vi "面积.vi"(8 "error in (no error)":errorcluster caption="错误输入（无错误）", 11 "矩形类 输入":refnum<class "矩形.lvclass"> caption="DNL_LabVIEW Object in") -> (0 "error out":errorcluster caption="错误输出", 2 "面积":dbl, 3 "矩形类 输出":refnum<class "矩形.lvclass"> caption="DNL_LabVIEW Object out")   [LabVIEW 2013, in "矩形.lvclass"]
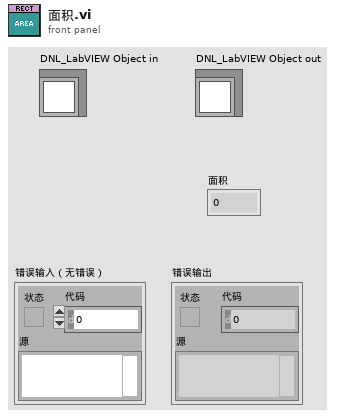
[diagram p1: front panel]
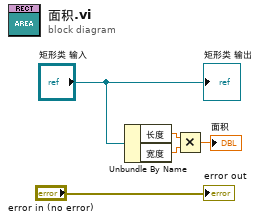
[diagram p0: block diagram]
diagram:
  n1 = Unbundle By Name("矩形类 输入") -> ("长度"=w3:dbl, "宽度"=w2:dbl)
  n2 = Multiply(x=w3, y=w2) -> (x*y=→"面积":dbl)
  "error out" <- "error in (no error)"
  "矩形类 输出" <- "矩形类 输入"
